vi "Sans titre 1.vi"() -> ()   [LabVIEW 2012]
panel:
  out "Booléen":bool
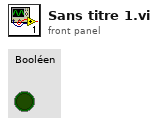
[diagram p1: front panel]
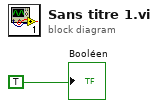
[diagram p0: block diagram]
diagram:
  "Booléen" <- TRUE
